vi "Judge Set Item Symbol.vi"(8 "error in (no error)":errorcluster, 9 "Symbol index":i32, 10 "Tag":string, 11 "TreeControl in":refnum<vi>) -> (0 "error out":errorcluster, 1 "Set out":T1, 2 "New Symbol Index":i32, 3 "TreeControl out":refnum<vi>, 5 "Set?":bool)   [LabVIEW 2023, in "DSLV_Tree.lvlib"]
uses:
  DSLV_Tree.lvlib
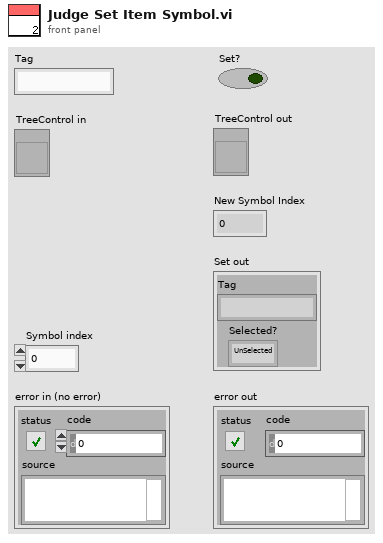
[diagram p1: front panel]
types:
  T1 = cluster{"Tag":string, "Selected?":enum16{"UnSelected", "Selected", "PartSelected"}}
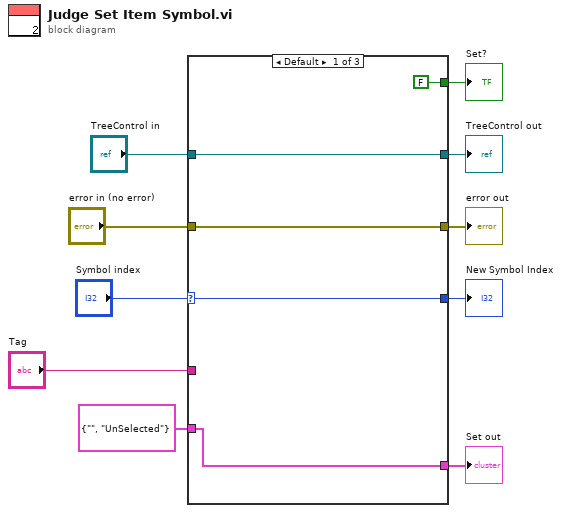
[diagram p0: block diagram]
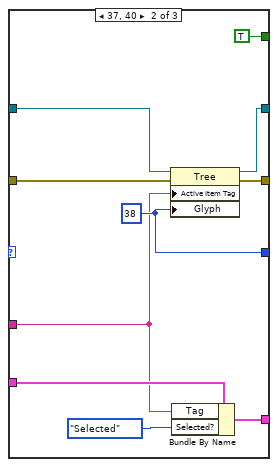
[diagram p2: hidden frame]
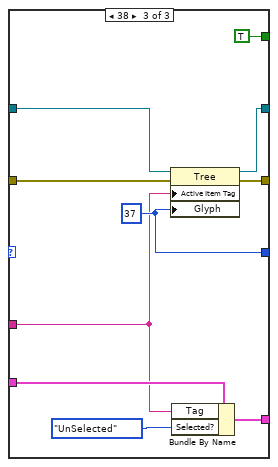
[diagram p3: hidden frame]
diagram:
  n1 = case shown="Default" "Symbol index" {
    selector: "Symbol index" -> [w13 _ _]
    tunnel: "TreeControl in" -> [w15 w25 w35]
    tunnel: "error in (no error)" -> [w14 w24 w34]
    tunnel: [w14 w23 w31] -> w3
    tunnel: [w15 w22 w32] -> w4
    tunnel: "Tag" -> [_ w18 w28]
    tunnel: [w11 w16 w26] -> w7
    tunnel: [FALSE TRUE TRUE] -> w8
    tunnel: [w13 w20 w30] -> w9
    tunnel: T1 {"Tag"="", "Selected?"=enum."UnSelected"} ("Set in") -> [w11 w19 w29]
    frame Default {
    }
    frame 37, 40 {
      w20 = 38 ("Active Item:Symbol Index")
      n2 = property on="Property Node" class="Tree"(reference=w25, error in=w24, "Active Item Tag"=w18, "Glyph"=w20) -> (reference out=w22:refnum<vi>, error out=w23:errorcluster)
      n3 = Bundle By Name(cluster=w19, "Tag"=w18, "Selected?"=enum16{"UnSelected", "Selected", "PartSelected"}."Selected") -> (w16:T1)
    }
    frame 38 {
      w30 = 37 ("Active Item:Symbol Index")
      n4 = property on="Property Node" class="Tree"(reference=w35, error in=w34, "Active Item Tag"=w28, "Glyph"=w30) -> (reference out=w32:refnum<vi>, error out=w31:errorcluster)
      n5 = Bundle By Name(cluster=w29, "Tag"=w28, "Selected?"=enum16{"UnSelected", "Selected", "PartSelected"}."UnSelected") -> (w26:T1)
    }
  }
  "New Symbol Index" <- w9
  "Set?" <- w8
  "Set out" <- w7
  "TreeControl out" <- w4
  "error out" <- w3
